vi "检查更新.vi"(8 "error in (no error)":errorcluster caption="错误输入（无错误）") -> (0 "error out":errorcluster, 2 "更新包名称":string)   [LabVIEW 2017]
uses:
  <vilib>/Utility/config.llb/Read Key (String).vi
  <vilib>/Utility/config.llb/NI_LVConfig.lvlib
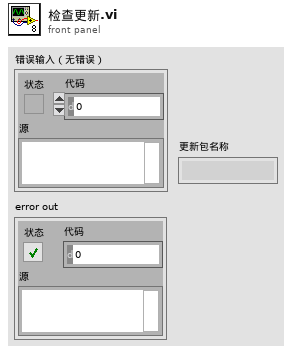
[diagram p1: front panel]
types:
  T1 = typedef "NI_LVConfig.lvlib/Config Data RefNum.ctl" = refnum<k1>
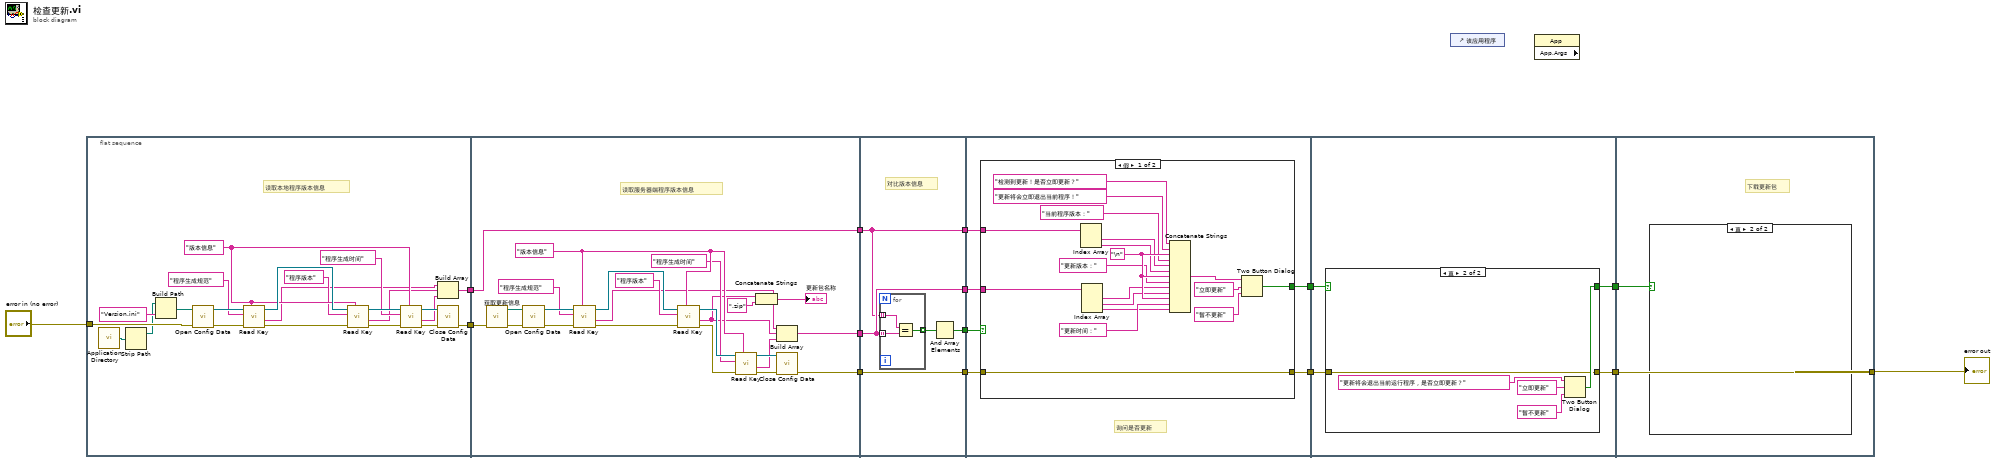
[diagram p0: block diagram]
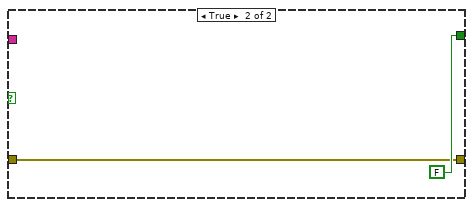
[diagram p2: hidden frame]
diagram:
  n1 = flat-sequence {
    tunnel: [w20] -> w15
    tunnel: [w19] -> w14
    tunnel: "error in (no error)" -> [w18]
    tunnel: w15 -> [w47]
    tunnel: w14 -> [w43]
    tunnel: [w43] -> w13
    tunnel: [w42] -> w12
    tunnel: [w41] -> w10
    tunnel: w13 -> [w61]
    tunnel: w12 -> [w62]
    tunnel: [w64] -> w11
    tunnel: w10 -> [w63]
    tunnel: [w63] -> w9
    tunnel: [w62] -> w8
    tunnel: [w61] -> w7
    tunnel: w11 -> [w74]
    tunnel: w9 -> [w70]
    tunnel: w8 -> [w73]
    tunnel: w7 -> [w72]
    tunnel: [w71] -> w6
    tunnel: [w69] -> w5
    tunnel: w6 -> [w98]
    tunnel: w5 -> [w96]
    tunnel: [w97] -> w2
    tunnel: [w95] -> w1
    tunnel: [w107] -> w4
    tunnel: w2 -> [w106]
    tunnel: w1 -> [w107]
    frame #0 {
      w28 = "版本信息" ("section")
      # "读取本地程序版本信息"
      n2 = call <vilib>:"Application Directory.vi"() -> ("Application Directory"=w17:path)
      n3 = Strip Path(path=w17) -> (stripped path=w16:path)  [unwired: 1 out]
      n4 = Build Path(base path=w16, name or relative path="Version.ini" ("名称或相对路径")) -> (appended path=w37:path)
      n5 = call <vilib>:"Open Config Data.vi"("error in (no error)"=w18, "configuration file path"=w37) -> ("error out"=w33:errorcluster, "refnum"=w36:T1)  [unwired: 7 in, 1 out]
      n6 = call-poly <vilib>:"Read Key.vi"("section"=w28, "error in (no error)"=w33, "key"="程序生成规范", "refnum"=w36) -> ("error out"=w32:errorcluster, "value"=w23:string, "refnum out"=w35:T1)  [unwired: 4 in, 1 out]
      n7 = call-poly <vilib>:"Read Key.vi"("section"=w28, "error in (no error)"=w32, "key"="程序版本", "refnum"=w35) -> ("error out"=w31:errorcluster, "value"=w22:string, "refnum out"=w34:T1)  [unwired: 4 in, 1 out]
      n8 = call-poly <vilib>:"Read Key.vi"("section"=w28, "error in (no error)"=w31, "key"="程序生成时间", "refnum"=w34) -> ("error out"=w29:errorcluster, "value"=w21:string, "refnum out"=w30:T1)  [unwired: 4 in, 1 out]
      n9 = Build Array(w23, w22, w21) -> (w19:string[])
      n10 = call <vilib>:"Close Config Data.vi"("error in (no error)"=w29, "refnum"=w30) -> ("error out"=w20:errorcluster)  [unwired: 8 in, 1 out]
    }
    frame #1 {
      w51 = "版本信息" ("section")
      # "读取服务器端程序版本信息"
      n11 = call "获取更新信息.vi"("error in (no error)"=w47) -> ("error out"=w46:errorcluster, "更新文件路径"=w60:path)  [unwired: 9 in]
      n12 = call <vilib>:"Open Config Data.vi"("error in (no error)"=w46, "configuration file path"=w60) -> ("error out"=w55:errorcluster, "refnum"=w52:T1)  [unwired: 7 in, 1 out]
      n13 = call-poly <vilib>:"Read Key.vi"("section"=w51, "error in (no error)"=w55, "key"="程序生成规范", "refnum"=w52) -> ("error out"=w56:errorcluster, "value"=w45:string, "refnum out"=w53:T1)  [unwired: 4 in, 1 out]
      n14 = call-poly <vilib>:"Read Key.vi"("section"=w51, "error in (no error)"=w56, "key"="程序版本", "refnum"=w53) -> ("error out"=w57:errorcluster, "value"=w40:string, "refnum out"=w54:T1)  [unwired: 4 in, 1 out]
      n15 = call-poly <vilib>:"Read Key.vi"("section"=w51, "error in (no error)"=w57, "key"="程序生成时间", "refnum"=w54) -> ("error out"=w59:errorcluster, "value"=w44:string, "refnum out"=w58:T1)  [unwired: 4 in, 1 out]
      n16 = Concatenate Strings(w40, ".zip" ("字符串")) -> (→"更新包名称":string)
      n17 = Build Array(w45, w40, w44) -> (w42:string[])
      n18 = call <vilib>:"Close Config Data.vi"("error in (no error)"=w59, "refnum"=w58) -> ("error out"=w41:errorcluster)  [unwired: 8 in, 1 out]
    }
    frame #2 {
      # "对比版本信息"
      n19 = for {
        tunnel: w61 -> [w66] mode=indexing
        tunnel: w62 -> [w68] mode=indexing
        tunnel: [w67] -> w65 mode=indexing
        n20 = Equal?(x=w66, y=w68) -> (x = y?=w67:bool)
      }
      n21 = And Array Elements(Boolean array=w65) -> (logical AND=w64:bool)
    }
    frame #3 {
      # "询问是否更新"
      n22 = case shown="假" w74 {
        tunnel: w73 -> [w85 _]
        tunnel: w72 -> [w84 _]
        tunnel: [w78 FALSE ("T button?")] -> w71
        tunnel: w70 -> [w77 w93]
        tunnel: [w77 w93] -> w69
        frame False {
          w91 = "\n"
          n23 = Index Array(array=w84) -> (element #1=w83:string, element #2=w82:string)  [unwired: 2 in]
          n24 = Index Array(array=w85) -> (element #1=w81:string, element #2=w80:string, element #3=w79:string)  [unwired: 3 in]
          n25 = Concatenate Strings("检测到更新！是否立即更新？" ("字符串"), "更新将会立即退出当前程序！" ("消息"), w91, "当前程序版本：" ("字符串"), w83, w82, w91, "更新版本：" ("字符串"), w81, w80, w91, "更新时间：" ("字符串"), w79) -> (w92:string)
          n26 = Two Button Dialog(message=w92, 1:"暂不更新" ("F按钮名称（“取消”）"), 2:"立即更新" ("T按钮名称（“确定”）")) -> (T button?=w78:bool)
        }
        frame True {
        }
      }
    }
    frame #4 {
      n27 = case shown="真" w98 {
        selector: w98 -> [w100 _]
        tunnel: [w100 w102] -> w97
        tunnel: [w99 w101] -> w95
        tunnel: w96 -> [w99 w101]
        frame False {
        }
        frame True {
          n28 = Two Button Dialog(message="更新将会退出当前运行程序，是否立即更新？" ("消息"), 1:"暂不更新" ("F按钮名称（“取消”）"), 2:"立即更新" ("T按钮名称（“确定”）")) -> (T button?=w102:bool)
        }
      }
    }
    frame #5 {
      # "下载更新包"
      n29 = case shown="真" w106 {
        frame False {
        }
        frame True {
        }
      }
    }
  }
  n30 = control-ref of="该应用程序"() -> ()  [unwired: 1 out]
  n31 = property class="App" props=["App.Args"]() -> ()  [unwired: 2 in, 3 out]
  "error out" <- w4
